vi "Tosca-Enumerate Required Endpoints.vi"(7 "Imaging":T1) -> (8 "Required Endpoints":cluster{string[]}[](array[cluster]))   [LabVIEW 2020]
uses:
  Typedefs/Tosca-Imaging.ctl
  Imaging VIs/Tosca-Imaging Mode.ctl
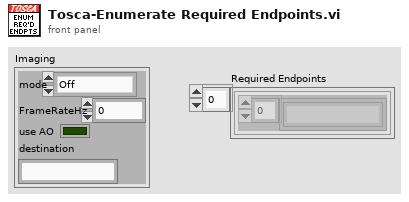
[diagram p1: front panel]
types:
  T1 = typedef "Tosca-Imaging.ctl" = cluster{"mode":T2, "FrameRateHz":dbl, "use AO":bool, "destination":string}
  T2 = typedef "Tosca-Imaging Mode.ctl" = enum16{"Off", "Widefield", "Two-photon"}
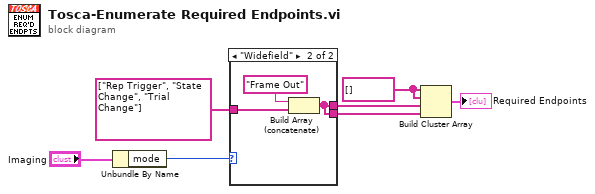
[diagram p0: block diagram]
diagram:
  w7 = string[] []
  n1 = Unbundle By Name("Imaging") -> ("mode"=w6:T2)
  n2 = case shown="\"Widefield\"" w6 {
    tunnel: string[] ["Rep Trigger", "State Change", "Trial Change"] -> [w8 w11]
    tunnel: [w8 w9] -> w2
    tunnel: [w8 w9] -> w1
    frame "Off", Default {
    }
    frame "Widefield" {
      n3 = Build Array (concatenate)("Frame Out", w11) -> (w9:string[])
    }
  }
  n4 = Build Cluster Array(w7, w7, w2, w1) -> (→"Required Endpoints":cluster{string[]}[])
